vi "LVProjectShortcut_AboutDialog.vi"(8 "error in (no error)":errorcluster) -> (0 "error out":errorcluster)   [LabVIEW 2017, in "LVProject Shortcut.lvlib"]
doc: "About dialog."
uses:
  LVProject Shortcut.lvlib
panel:
  out "String Indicator":string
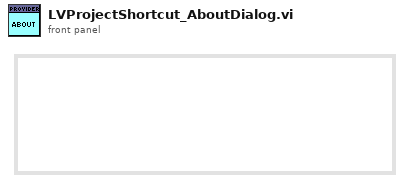
[diagram p1: front panel]
types:
  T1 = cluster{"Version String":string, "Name":string, "Copyright":string, "License":string}
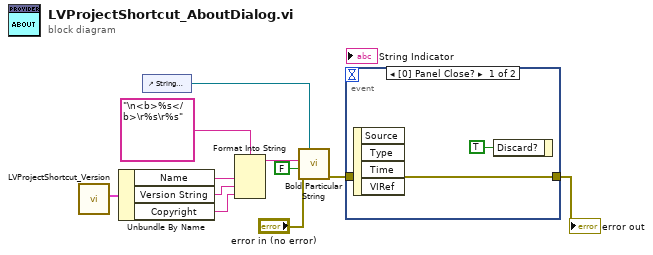
[diagram p0: block diagram]
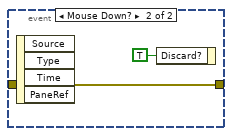
[diagram p2: hidden frame]
diagram:
  n1 = call "LVProjectShortcut_Version.vi"() -> ("Library Info"=w11:T1)  [unwired: 11 in]
  n2 = Unbundle By Name(w11) -> ("Name"=w10:string, "Version String"=w9:string, "Copyright"=w8:string)
  n3 = control-ref of="String Indicator"() -> (w5:refnum<vi>)
  n4 = Format Into String(format string="\n<b>%s</b>\r%s\r%s", w10, w9, w8) -> (resulting string=w6:string)  [unwired: 2 in, 1 out]
  n5 = call <vilib>:"Bold Particular String.vi"("error in (no error)"="error in (no error)", "resize string? (TRUE)"=FALSE, "text to display"=w6, "string refnum"=w5) -> ("error out"=w3:errorcluster)  [unwired: 6 in, 1 out]
  n6 = event shown="[0] Panel Close?" {
    selector: _ -> [_ _]
    dyn-events: _ -> [_ _]
    timeout: _ -> [_ _]
    tunnel: w3 -> [w12 w14]
    tunnel: [w12 w14] -> w1
    event Panel Close? {
      n7 = event-data() -> ()  [unwired: 1 in, 4 out]
      n8 = event-data("Discard?"=TRUE) -> ()  [unwired: 1 in, 1 out]
    }
    event Mouse Down? {
      n9 = event-data() -> ()  [unwired: 1 in, 4 out]
      n10 = event-data("Discard?"=TRUE) -> ()  [unwired: 1 in, 1 out]
    }
  }
  "error out" <- w1
